vi "motorInit.vi"(1 "电机步进":dbl=5.0, 2 "电机长度":dbl=200.0) -> (0 "电机移动次数":dbl format="%#_13g")   [LabVIEW 2018]
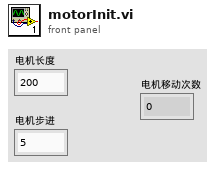
[diagram p1: front panel]
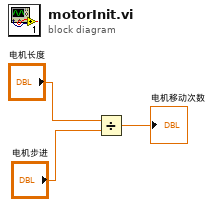
[diagram p0: block diagram]
diagram:
  n1 = Divide(x="电机长度", y="电机步进") -> (x/y=→"电机移动次数":dbl)
